vi "Main Page.vi"(8 "error in (no error)":errorcluster, 11 "Node Ptr":T1 format="%.0x") -> (0 "error out":errorcluster)   [LabVIEW 2019, in "Fuel Injector Analysis Addon System Explorer.lvlib"]
uses:
  Fuel Injector Analysis Addon System Explorer.lvlib
  <vilib>/NI VeriStand/Custom Device API/Custom Device API.lvlib
  Addon Shared/Fuel Injector Analysis Addon Shared.lvlib
  Addon Shared/SubVIs/Constants.vi
  <vilib>/NI VeriStand/Custom Device API/Set Item Property (String).vi
  <vilib>/NI/NI VeriStand Hardware Resource Discovery/NIVS Hardware Discovery.lvlib
  <vilib>/NI/NI VeriStand Hardware Resource Discovery/_Types/Filter Type.ctl
  <vilib>/NI VeriStand/Custom Device API/Custom Device Item Ref.ctl
panel:
  out "Version":string
  in  "RIO Browse":bool
  in  "SHDocVw.IWebBrowser":refnum<k7>(container)
  in  "Description":string
  in  "RIO Device":string
  in  "Local Bitfile path":path
  in  "Header":cluster{"Section Name":string}={"Section Name"="Custom Device Item Settings"}
  in  "Name":string
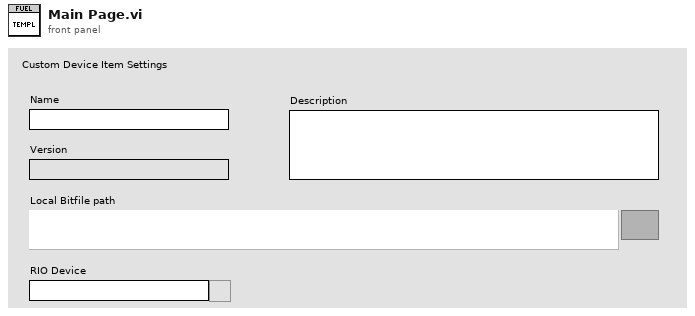
[diagram p1: front panel]
types:
  T1 = typedef "Custom Device API.lvlib/Custom Device Item Ref.ctl" = u64
  T2 = typedef "Custom Device API.lvlib/Custom Device Item Info.ctl" = cluster{"Name":string, "Is Channel":bool, "GUID":string, "Is Waveform":bool}
  T3 = typedef "Fuel Injector Analysis Addon Shared.lvlib/Main Settings.ctl" = cluster{"RIO Device Address":string, "Local bitfile path":path, "RT bitfile path":path, "Number of injectors":u16}
  T4 = typedef "NIVS Hardware Discovery.lvlib/Filter Type.ctl" = enum16{"Device Category", "Product Name", "Ethernet", "XNET", "VISA", "FPGA", "EtherCAT Master", "DAQmx", "GPIB", "Serial"}
  T5 = enum16{"0", "1", "2", "3", "4", "5", "6", "7", "8"}
  T6 = typedef "Custom Device API.lvlib/Custom Device Commands.ctl" = enum16{"Default", "Item renamed", "Shutdown", "Dynamic button pressed"}
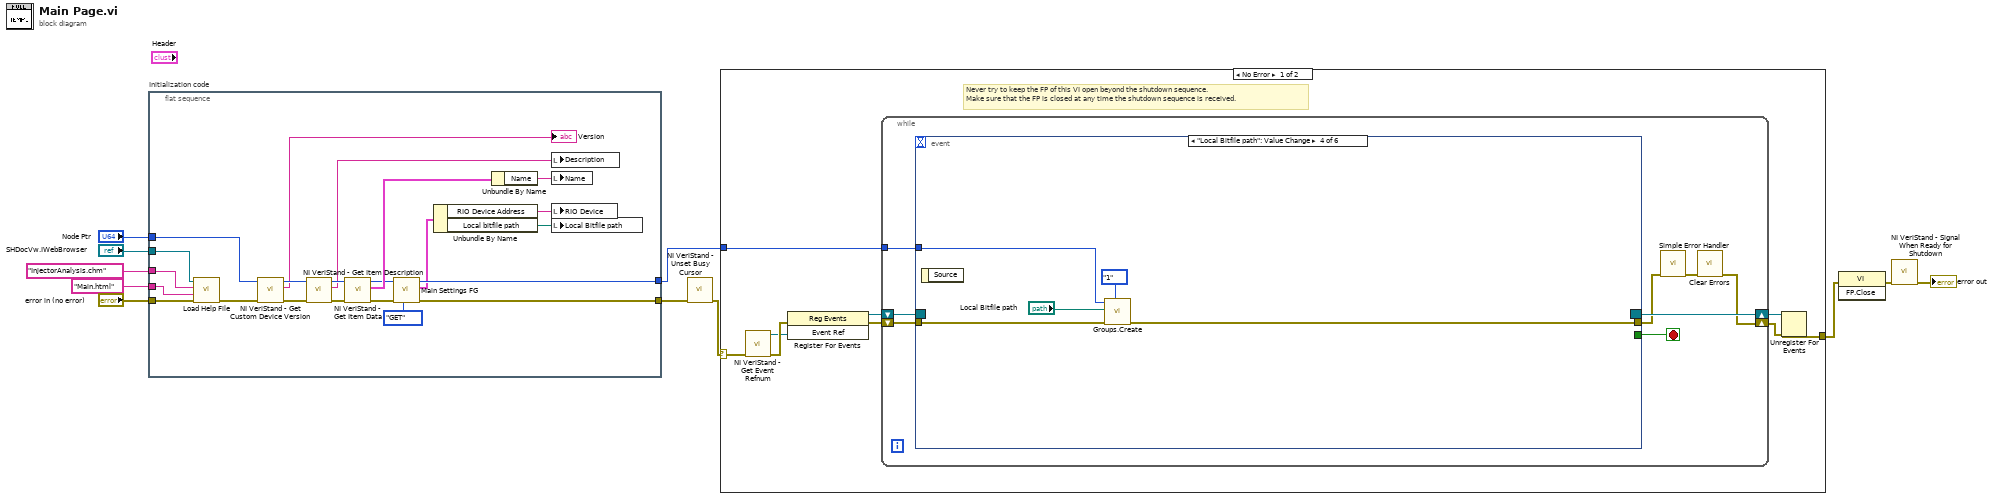
[diagram p0: block diagram]
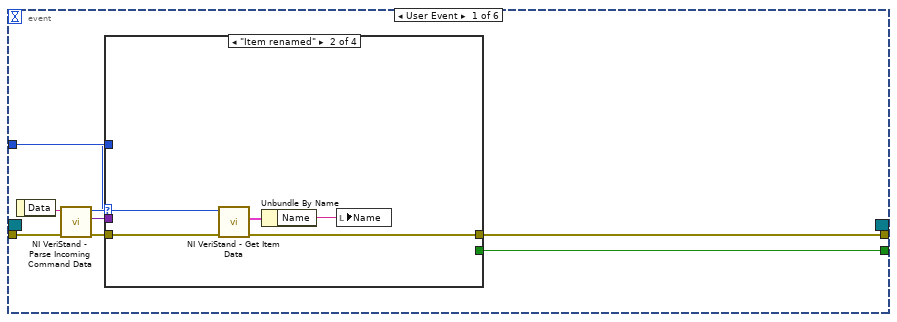
[diagram p2: hidden frame]
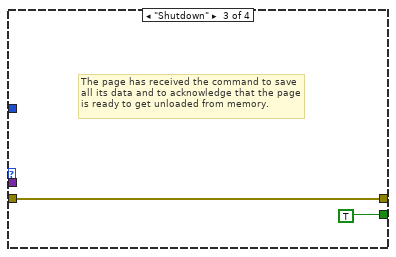
[diagram p4: hidden frame]
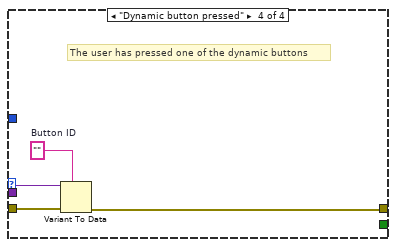
[diagram p5: hidden frame]
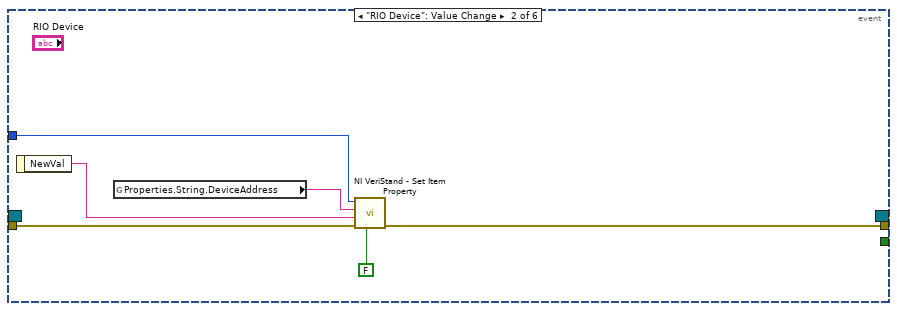
[diagram p6: hidden frame]
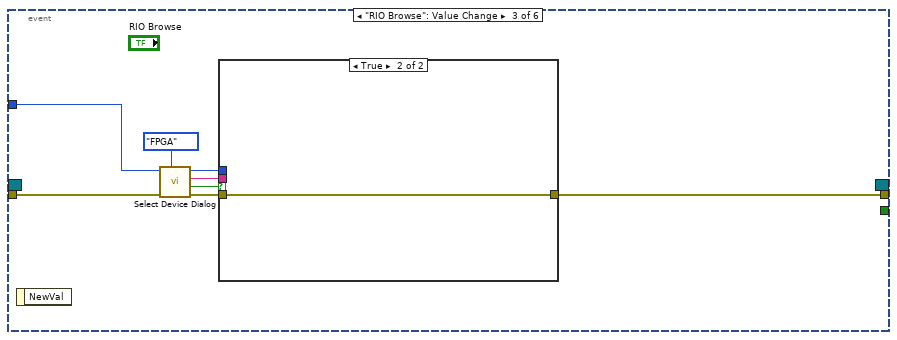
[diagram p7: hidden frame]
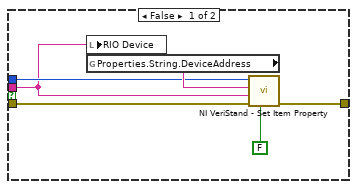
[diagram p8: hidden frame]
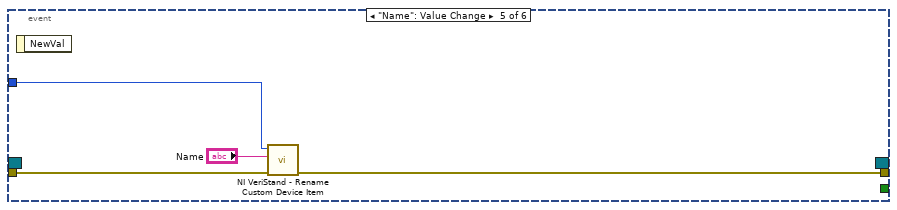
[diagram p9: hidden frame]
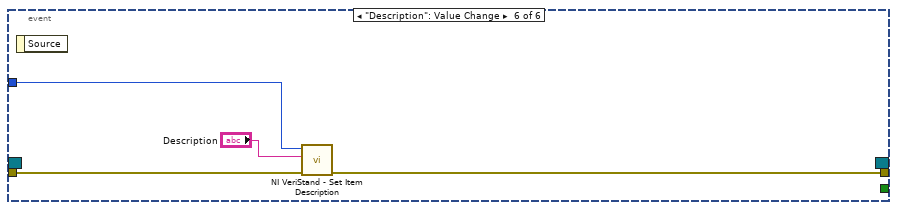
[diagram p10: hidden frame]
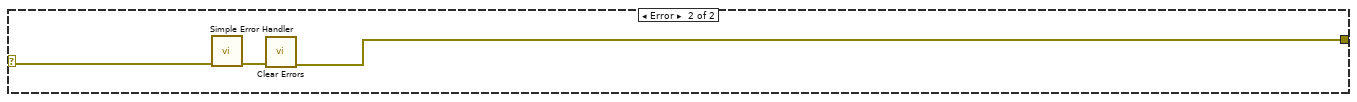
[diagram p11: hidden frame]
diagram:
  n1 = flat-sequence "Initialization code" {
    tunnel: "error in (no error)" -> [w21]
    tunnel: "Node Ptr" -> [w13]
    tunnel: [w17] -> w7
    tunnel: [w27] -> w4
    tunnel: "Main.html" ("HTML File") -> [w20]
    tunnel: "InjectorAnalysis.chm" ("Main CHM File") -> [w19]
    tunnel: "SHDocVw.IWebBrowser" -> [w18]
    frame #0 {
      n2 = call "Load Help File.vi"("error in (no error)"=w21, "HTML File"=w20, "Main CHM File"=w19, "SHDocVw.IWebBrowser2"=w18) -> ("error out"=w16:errorcluster)  [unwired: 7 in]
      n3 = call <vilib>:"NI VeriStand - Get Custom Device Version.vi"("error in (no error)"=w16, "Device Ref in"=w13) -> ("error out"=w15:errorcluster, "Value"=→"Version":string, "Device Ref out"=w14:T1)  [unwired: 7 in]
      n4 = call <vilib>:"NI VeriStand - Get Item Description.vi"("error in (no error)"=w15, "Item Ref in"=w14) -> ("error out"=w32:errorcluster, "Description"=w22:string, "Item Ref out"=w33:T1)  [unwired: 7 out]
      n5 = call <vilib>:"NI VeriStand - Get Item Data.vi"("error in (no error)"=w32, "Item Ref in"=w33) -> ("error out"=w29:errorcluster, "Item Info"=w31:T2, "Item Ref out"=w28:T1)  [unwired: 7 out]
      n6 = call "Main Settings FG.vi"("Action"=enum8{"GET", "SET"}."GET", "error in (no error)"=w29, "Item Ref"=w28) -> ("error out"=w17:errorcluster, "Main Settings out"=w25:T3, "Item Ref out"=w27:T1)  [unwired: 6 in]
      n7 = Unbundle By Name(w25) -> ("RIO Device Address"=w24:string, "Local bitfile path"=w23:path)
      n8 = Unbundle By Name(w31) -> ("Name"=w30:string)
      n9 = local write "Description"(w22) -> ()
      n10 = local write "Name"(w30) -> ()
      n11 = local write "RIO Device"(w24) -> ()
      n12 = local write "Local Bitfile path"(w23) -> ()
    }
  }
  n13 = call <vilib>:"NI VeriStand - Unset Busy Cursor.vi"("error in (no error)"=w7) -> ("error out"=w6:errorcluster)  [unwired: 10 out]
  n14 = case shown="No Error" w6 {
    selector: w6 -> [w34 w107]
    tunnel: [w39 w105] -> w11
    tunnel: w4 -> [w35 _]
    frame No Error {
      # "Never try to keep the FP of this VI open beyond the shutdown sequence.\nMake sure that the FP is closed at any time the shutdown sequence is received."
      n15 = call <vilib>:"NI VeriStand - Get Event Refnum.vi"("error in (no error)"=w34) -> ("error out"=w42:errorcluster, "Event Ref"=w38:refnum<user-event>)  [unwired: 9 out]
      n16 = register-events(error in=w42, w38) -> (reference out=w36:refnum<event-registration>, error out=w37:errorcluster)  [unwired: 1 in]
      n17 = while {
        tunnel: w35 -> [w46]
        shift-right: [w43] -> w40
        shift-left: w37 -> [w49]
        shift-right: [w50] -> w41
        shift-left: w36 -> [w48]
        stop <- w47 stop-if-true
        n18 = event shown="[3] \"Local Bitfile path\": Value Change" {
          selector: w48 -> [_ _ _ _ _ _]
          dyn-events: [_ _ _ _ _ _] -> w50
          timeout: _ -> [_ _ _ _ _ _]
          tunnel: w49 -> [w58 w76 w83 w94 w100 w104]
          tunnel: [w54 _ _ _ _ _] -> w47
          tunnel: [w53 w72 w84 w96 w99 w101] -> w45
          tunnel: w46 -> [w52 w73 w81 w93 w98 w103]
          event User Event {
            n19 = event-data() -> ("Data"=w57:string)  [unwired: 1 out]
            n20 = call <vilib>:"NI VeriStand - Parse Incoming Command Data.vi"("error in (no error)"=w58, "Incoming data"=w57) -> ("error out"=w56:errorcluster, "Outgoing data"=w51:variant, "Action"=w55:T6)  [unwired: 7 out]
            n21 = case shown="\"Item renamed\"" w55 {
              tunnel: w56 -> [w59 w64 w65 w70]
              tunnel: [_ _ TRUE _] -> w54
              tunnel: [w59 w61 w65 w67] -> w53
              tunnel: w52 -> [_ w63 _ _]
              tunnel: w51 -> [_ _ _ w69]
              frame "Default", Default {
              }
              frame "Item renamed" {
                n22 = call <vilib>:"NI VeriStand - Get Item Data.vi"("error in (no error)"=w64, "Item Ref in"=w63) -> ("error out"=w61:errorcluster, "Item Info"=w62:T2)  [unwired: 8 out]
                n23 = Unbundle By Name(w62) -> ("Name"=w60:string)
                n24 = local write "Name"(w60) -> ()
              }
              frame "Shutdown" {
                # "The page has received the command to save all its data and to acknowledge that the page is ready to get unloaded from memory."
              }
              frame "Dynamic button pressed" {
                w68 = ""  # Button ID
                # "The user has pressed one of the dynamic buttons"
                n25 = Variant To Data(error in=w70, type=w68, Variant=w69) -> (error out=w67:errorcluster)  [unwired: 1 out]
              }
            }
          }
          event "RIO Device": Value Change {
            n26 = event-data() -> ("NewVal"=w75:string)  [unwired: 1 out]
            n27 = global read "Constants.vi" "Properties.String.DeviceAddress"() -> (w74:string)
            n28 = call-poly <vilib>:"NI VeriStand - Set Item Property.vi"("Binary String (T)"=FALSE, "error in (no error)"=w76, "Value"=w75, "Property Name"=w74, "Item Ref in"=w73) -> ("error out"=w72:errorcluster)  [unwired: 4 in, 2 out]
          }
          event "RIO Browse": Value Change {
            n29 = event-data() -> ()  [unwired: 2 out]
            n30 = call <vilib>:"Select Device Dialog.vi"("Filter Type"=Filter_Type."FPGA", "error in (no error)"=w83, "Item Ref in"=w81) -> ("error out"=w82:errorcluster, "Cancelled?"=w79:bool, "Selected Alias"=w78:string, "Item Ref out"=w80:T1)  [unwired: 5 in]
            n31 = case shown="True" w79 {
              tunnel: w82 -> [w90 w91]
              tunnel: w80 -> [w88 _]
              tunnel: [w87 w91] -> w84
              tunnel: w78 -> [w85 _]
              frame False {
                n32 = local write "RIO Device"(w85) -> ()
                n33 = global read "Constants.vi" "Properties.String.DeviceAddress"() -> (w89:string)
                n34 = call-poly <vilib>:"NI VeriStand - Set Item Property.vi"("Binary String (T)"=FALSE, "error in (no error)"=w90, "Value"=w85, "Property Name"=w89, "Item Ref in"=w88) -> ("error out"=w87:errorcluster)  [unwired: 4 in, 2 out]
              }
              frame True {
              }
            }
          }
          event "Local Bitfile path": Value Change {
            n35 = event-data() -> ()  [unwired: 2 out]
            n36 = call "Groups.Create.vi"("Max Shots"=T5."1", "error in (no error)"=w94, "NewVal"="Local Bitfile path", "Item Ref in"=w93) -> ("error out"=w96:errorcluster)  [unwired: 6 in, 1 out]
          }
          event "Name": Value Change {
            n37 = event-data() -> ()  [unwired: 2 out]
            n38 = call <vilib>:"NI VeriStand - Rename Custom Device Item.vi"("error in (no error)"=w100, "New Name"="Name", "Item Ref in"=w98) -> ("error out"=w99:errorcluster)  [unwired: 1 in, 7 out]
          }
          event "Description": Value Change {
            n39 = event-data() -> ()  [unwired: 2 out]
            n40 = call <vilib>:"NI VeriStand - Set Item Description.vi"("error in (no error)"=w104, "Description"="Description", "Item Ref in"=w103) -> ("error out"=w101:errorcluster)  [unwired: 6 in, 2 out]
          }
        }
        n41 = call <vilib>:"Simple Error Handler.vi"("error in (no error)"=w45) -> ("error out"=w44:errorcluster)  [unwired: 1 in, 7 out]
        n42 = call <vilib>:"Clear Errors.vi"("error in (no error)"=w44) -> ("error out"=w43:errorcluster)  [unwired: 1 in, 5 out]
      }
      n43 = Unregister For Events(event registration refnum=w41, error in=w40) -> (error out=w39:errorcluster)
    }
    frame Error {
      n44 = call <vilib>:"Simple Error Handler.vi"("error in (no error)"=w107) -> ("error out"=w106:errorcluster)  [unwired: 1 in, 7 out]
      n45 = call <vilib>:"Clear Errors.vi"("error in (no error)"=w106) -> ("error out"=w105:errorcluster)  [unwired: 1 in, 5 out]
    }
  }
  n46 = invoke class="VI" method="FP.Close"(error in=w11) -> (error out=w10:errorcluster)  [unwired: 2 in, 2 out]
  n47 = call <vilib>:"NI VeriStand - Signal When Ready for Shutdown.vi"("error in (no error)"=w10) -> ("error out"=→"error out":errorcluster)  [unwired: 10 out]
